vi "Climber Controller.vi"(8 "error in":errorcluster) -> ()   [LabVIEW 2019]
doc: "This VI executes continuously carrying out the current operation and responding to updates or new operations. It will often contain the timing or control code that is difficult to place directly in TeleOp. This VI generally opens all sensors and motors and isolates the rest of the robot code from knowing how the operations are carried out."
uses:
  Climber Setpoints.ctl
  Climber Operations.ctl
  <vilib>/Rock Robotics/WPI/Solenoid/WPI_SolenoidChannel.ctl
  <vilib>/Rock Robotics/WPI/Solenoid/WPI_SolenoidValue.ctl
  <vilib>/Rock Robotics/WPI/ThirdParty/Phoenix-LabVIEW/Motor Controller/Controls/CTRE_Phoenix_MotorControl_ControlMode.ctl
  <vilib>/Rock Robotics/WPI/ThirdParty/Phoenix-LabVIEW/Motor Controller/Controls/CTRE_Phoenix_MotorControl_NeutralMode.ctl
  <vilib>/Rock Robotics/WPI/Solenoid/WPI_SolenoidOpenSingle.vi
  <vilib>/Rock Robotics/WPI/Solenoid/WPI_SolenoidSetEnum.vi
  <vilib>/addons/control/pid/pid.llb/PID (DBL).vi
  <vilib>/Rock Robotics/Network Tables/NT Write Boolean.vi
  <vilib>/addons/control/pid/NI_PID_pid.lvlib
panel:
  out "Current\nCmd":string
  # "Tip: It may be helpful to observe inputs and sensor values.\nYou may also want to display tuning or debugging controls."
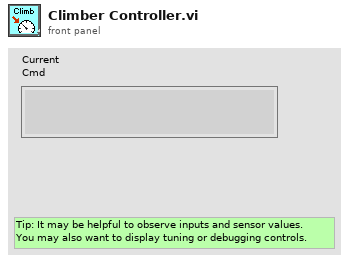
[diagram p1: front panel]
types:
  T1 = typedef "CTRE_Phoenix_MotorControl_NeutralMode.ctl" = enum8{"EEPROMSetting", "Override to Coast", "Override to Brake"}
  T2 = typedef "CTRE_Phoenix_MotorControl_ControlMode.ctl" = u16
  T3 = typedef "WPI_SolenoidValue.ctl" = enum16{"Off", "On", "Forward", "Reverse"}
  T4 = typedef "WPI_SolenoidChannel.ctl" = enum8{"Solenoid 0", "Solenoid 1", "Solenoid 2", "Solenoid 3", "Solenoid 4", "Solenoid 5", "Solenoid 6", "Solenoid 7", "Invalid"}
  T5 = typedef "Climber Setpoints.ctl" = cluster{"Operation":T6, "Setpoint":dbl, "Duration":dbl}
  T6 = typedef "Climber Operations.ctl" = enum16{"Reserve", "Read Current", "Immediate", "Up", "Down", "Position Auto", "Position Manual"}
  T7 = typedef "WPI_MotorControlDeviceRef.ctl" = cluster{"DeviceStatus":errorcluster, "Type":T8, "PWM":cluster{"PWM Channel":T9, "DeadBand":T10}, "CAN":cluster{"Device Number":u8, "SetOutput VI Ref":variant, "GetOutput VI Ref":variant, "Enable VI Ref":variant, "Disable VI Ref":variant, "Data":variant}, "Invert":bool, "DIO PWM":cluster{"PWM \"Enable\" Channel":T9, "DIOChannel":T11, "PWM Rate":dbl}}
  T8 = typedef "WPI_MotorControlType.ctl" = enum16{"PWM", "CAN", "DIO PWM"}
  T9 = typedef "FPGA_DIOPWMChannel.ctl" = enum8{"PWM 0", "PWM 1", "PWM 2", "PWM 3", "PWM 4", "PWM 5", "PWM 6", "PWM 7", "PWM 8", "PWM 9", "PWM MXP 0", "PWM MXP 1", "PWM MXP 2", "PWM MXP 3", "PWM MXP 4", "PWM MXP 5", "PWM MXP 6", "PWM MXP 7", "PWM MXP 8", "PWM MXP 9", "Invalid"}
  T10 = typedef "WPI_PWMDeadband.ctl" = cluster{"Name":string, "maxPositivePwm":i32, "minPositivePwm":i32, "centerPwm":i32, "maxNegativePwm":i32, "minNegativePwm":i32, "angularRange":u16}
  T11 = typedef "FPGA_DIOChannel.ctl" = enum8{"DIO 0", "DIO 1", "DIO 2", "DIO 3", "DIO 4", "DIO 5", "DIO 6", "DIO 7", "DIO 8", "DIO 9", "DIO MXP 0", "DIO MXP 1", "DIO MXP 2", "DIO MXP 3", "DIO MXP 4", "DIO MXP 5", "DIO MXP 6", "DIO MXP 7", "DIO MXP 8", "DIO MXP 9", "DIO MXP 10", "DIO MXP 11", "DIO MXP 12", "DIO MXP 13", "DIO MXP 14", "DIO MXP 15", "SPI Port CS1", "SPI Port CS2", "SPI Port CS3", "SPI Port MISO", "SPI Port MOSI", "Invalid"}
  T12 = typedef "WPI_SolenoidDevRef.ctl" = cluster{"DevStatus":errorcluster, "Pneumatics Control Module":u8, "Forward Solenoid Channel":T4, "Reverse Solenoid Channel":T4}
  T13 = typedef "Command Status Info.ctl" = cluster{"Name":string, "Status":T14, "notifier out":T15}
  T14 = typedef "Completion Status.ctl" = enum16{"Successful", "Aborted", "Incomplete"}
  T15 = typedef "Completion Notifier.ctl" = refnum<notifier>
  T16 = cluster{"Current Command":T5, "Command Timing":cluster{"Start Time (ms)":u32, "Iterations":i32}, "Command Arguments":cluster{"Command Info":T13, "Description":string, "Default Command":T5, "queue out":refnum<queue>, "Subsystem Name":string}}
  T17 = cluster{"proportional gain (Kc)":dbl, "integral time (Ti, min)":dbl, "derivative time (Td, min)":dbl}
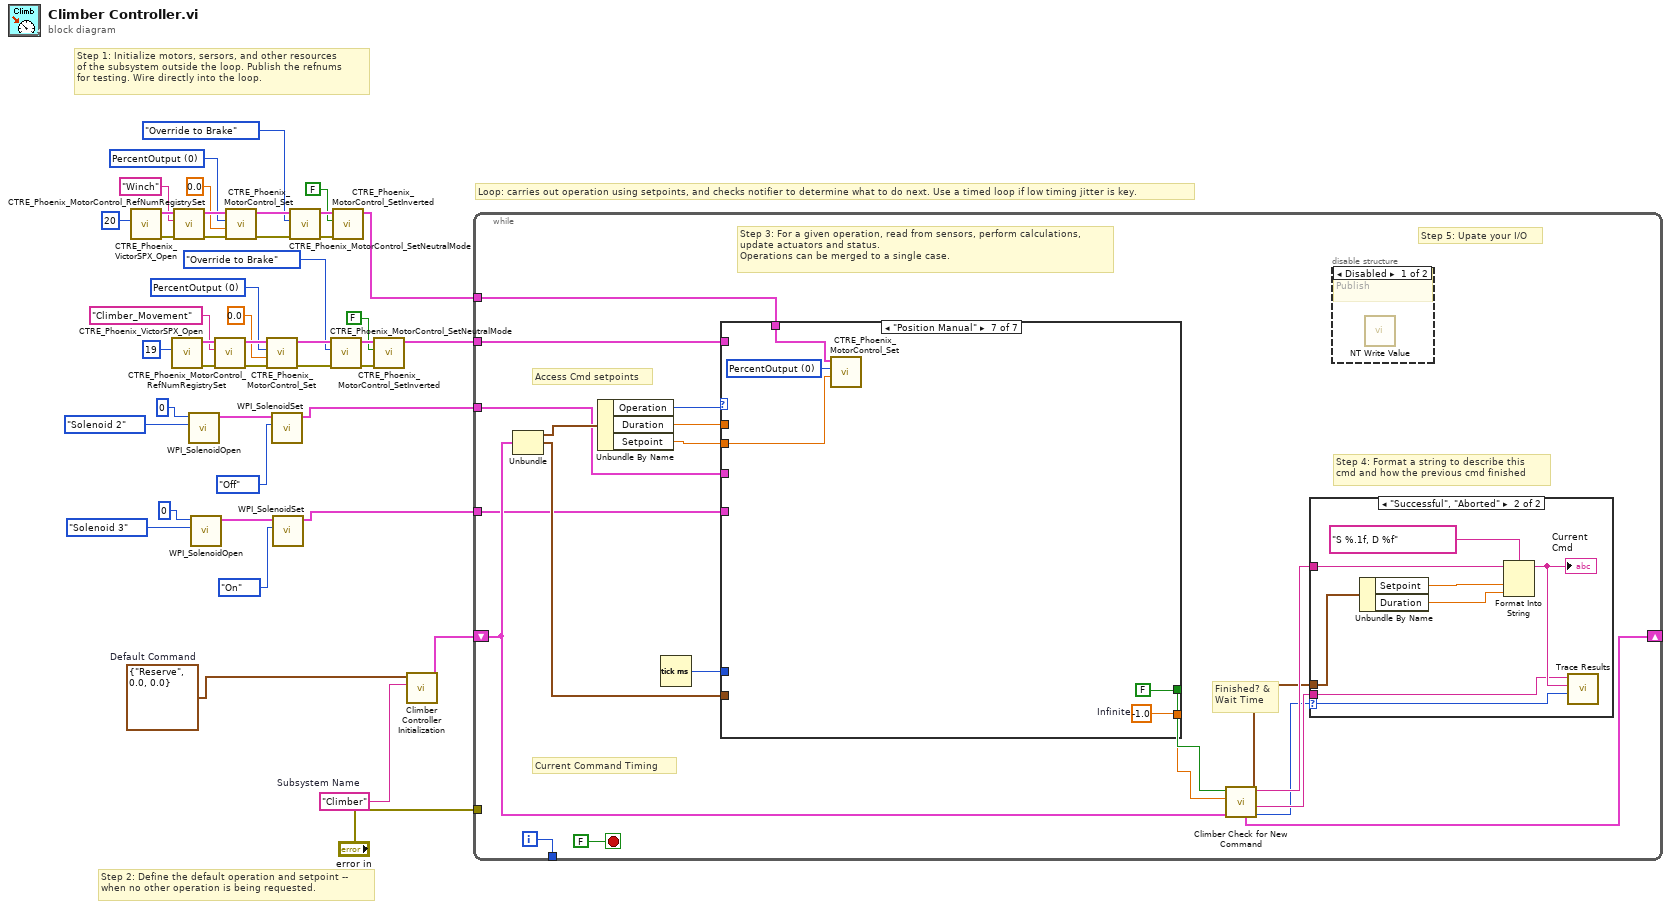
[diagram p0: block diagram]
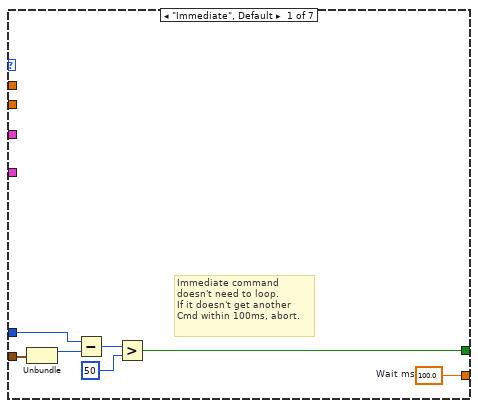
[diagram p4: hidden frame]
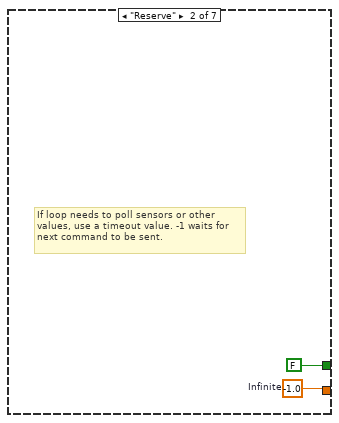
[diagram p5: hidden frame]
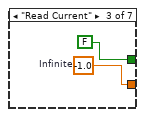
[diagram p6: hidden frame]
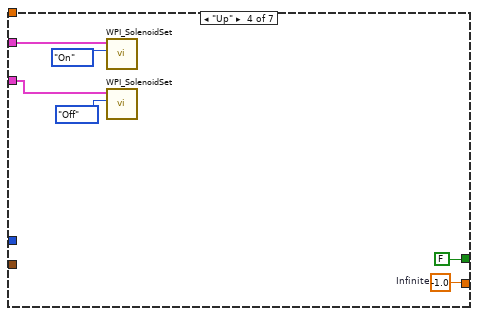
[diagram p7: hidden frame]
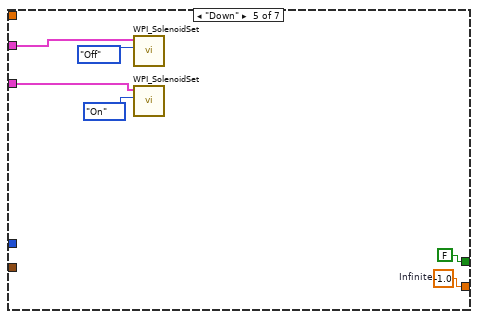
[diagram p8: hidden frame]
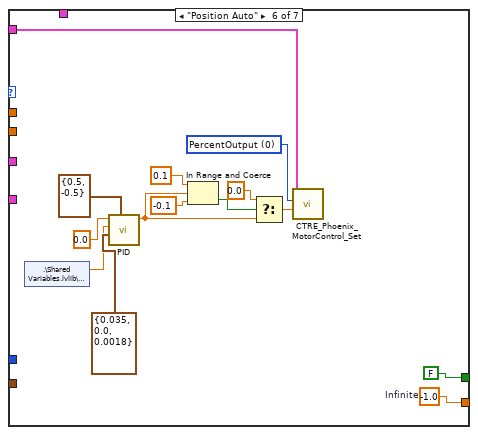
[diagram p9: hidden frame]
diagram:
  w6 = T2 0 items=["PercentOutput"=0, "Position"=1, "Velocity"=2, "Current"=3, "Follower"=5, "MotionProfile"=6, "MotionMagic"=7, "MotionProfileArc"=10, "Disabled"=15] ("Control Mode")
  w31 = T2 0 items=["PercentOutput"=0, "Position"=1, "Velocity"=2, "Current"=3, "Follower"=5, "MotionProfile"=6, "MotionMagic"=7, "MotionProfileArc"=10, "Disabled"=15] ("Control Mode")
  w41 = T5 {"Operation"=enum."Reserve", "Setpoint"=0.0, "Duration"=0.0}  # Default Command
  w42 = "Climber"  # Subsystem Name
  # "Step 2: Define the default operation and setpoint --\nwhen no other operation is being requested."
  # "Step 1: Initialize motors, sersors, and other resources\nof the subsystem outside the loop. Publish the refnums\nfor testing. Wire directly into the loop."
  # "Loop: carries out operation using setpoints, and checks notifier to determine what to do next. Use a timed loop if low timing jitter is key."
  n1 = call <vilib>:"CTRE_Phoenix_VictorSPX_Open.vi"("Device Number"=u8 20) -> ("error out"=w8:errorcluster, "CAN Talon SRX Ref"=w15:T7)  [unwired: 9 in]
  n2 = call <vilib>:"CTRE_Phoenix_VictorSPX_Open.vi"("Device Number"=u8 19) -> ("error out"=w33:errorcluster, "CAN Talon SRX Ref"=w40:T7)  [unwired: 9 in]
  n3 = call <vilib>:"CTRE_Phoenix_MotorControl_RefNumRegistrySet.vi"("error in (no error)"=w8, "refnum name"="Winch", "PhoenixMotorControlDevRef"=w15) -> ("error out"=w9:errorcluster, "PhoenixMotorControlDevRef"=w14:T7)  [unwired: 7 in]
  n4 = call-poly <vilib>:"WPI_SolenoidOpen.vi"("Solenoid Channel"=WPI_SolenoidChannel."Solenoid 2", "Pneumatics Control Module (0)"=u8 0) -> ("SolenoidDevRef"=w18:T12)  [unwired: 8 in, 1 out]
  n5 = call-poly <vilib>:"WPI_SolenoidOpen.vi"("Solenoid Channel"=WPI_SolenoidChannel."Solenoid 3", "Pneumatics Control Module (0)"=u8 0) -> ("SolenoidDevRef"=w16:T12)  [unwired: 8 in, 1 out]
  n6 = call <vilib>:"CTRE_Phoenix_MotorControl_RefNumRegistrySet.vi"("error in (no error)"=w33, "refnum name"="Climber_Movement", "PhoenixMotorControlDevRef"=w40) -> ("error out"=w34:errorcluster, "PhoenixMotorControlDevRef"=w39:T7)  [unwired: 7 in]
  n7 = call <vilib>:"CTRE_Phoenix_MotorControl_Set.vi"("error in (no error)"=w9, "Output"=0.0, "Control Mode"=w6, "PhoenixMotorControlDevRef"=w14) -> ("error out"=w10:errorcluster, "PhoenixMotorControlDevRef"=w13:T7)  [unwired: 6 in]
  n8 = call <vilib>:"CTRE_Phoenix_MotorControl_Set.vi"("error in (no error)"=w34, "Output"=0.0, "Control Mode"=w31, "PhoenixMotorControlDevRef"=w39) -> ("error out"=w35:errorcluster, "PhoenixMotorControlDevRef"=w38:T7)  [unwired: 6 in]
  n9 = call-poly <vilib>:"WPI_SolenoidSet.vi"("Value"=WPI_SolenoidValue."Off", "SolenoidDevRef"=w18) -> ("SolenoidDevRef"=w19:T12)  [unwired: 8 in, 1 out]
  n10 = call-poly <vilib>:"WPI_SolenoidSet.vi"("Value"=WPI_SolenoidValue."On", "SolenoidDevRef"=w16) -> ("SolenoidDevRef"=w17:T12)  [unwired: 8 in, 1 out]
  n11 = call <vilib>:"CTRE_Phoenix_MotorControl_SetNeutralMode.vi"("error in (no error)"=w10, "Motor Control Neutral Mode"=CTRE_Phoenix_MotorControl_NeutralMode."Override to Brake", "PhoenixMotorControlDevRef"=w13) -> ("error out"=w11:errorcluster, "PhoenixMotorControlDevRef"=w12:T7)  [unwired: 7 in]
  n12 = call <vilib>:"CTRE_Phoenix_MotorControl_SetNeutralMode.vi"("error in (no error)"=w35, "Motor Control Neutral Mode"=CTRE_Phoenix_MotorControl_NeutralMode."Override to Brake", "PhoenixMotorControlDevRef"=w38) -> ("error out"=w36:errorcluster, "PhoenixMotorControlDevRef"=w37:T7)  [unwired: 7 in]
  n13 = call <vilib>:"CTRE_Phoenix_MotorControl_SetInverted.vi"("error in (no error)"=w11, "Invert?"=FALSE, "PhoenixMotorControlDevRef"=w12) -> ("PhoenixMotorControlDevRef"=w1:T7)  [unwired: 7 in, 1 out]
  n14 = call <vilib>:"CTRE_Phoenix_MotorControl_SetInverted.vi"("error in (no error)"=w36, "Invert?"=FALSE, "PhoenixMotorControlDevRef"=w37) -> ("PhoenixMotorControlDevRef"=w26:T7)  [unwired: 7 in, 1 out]
  n15 = call "Climber Controller Initialization.vi"("Subsystem Name"=w42, "Default Command"=w41) -> ("Current Command"=w43:T16)  [unwired: 9 in]
  n16 = while {
    shift-right: [w56] -> _
    shift-left: w43 -> [w49]
    tunnel: [w63] -> _
    tunnel: "error in" -> [_]
    tunnel: w26 -> [w48]
    tunnel: w17 -> [w47]
    tunnel: w19 -> [w46]
    tunnel: w1 -> [w45]
    i -> [w63]
    stop <- FALSE stop-if-true
    # "Step 5: Upate your I/O"
    # "Step 4: Format a string to describe this\ncmd and how the previous cmd finished"
    # "Current Command Timing"
    # "Access Cmd setpoints"
    # "Finished? &\nWait Time"
    # "Step 3: For a given operation, read from sensors, perform calculations,\nupdate actuators and status.\nOperations can be merged to a single case."
    n17 = Unbundle(w49) -> ("Current Command"=w62:T5, "Command Timing"=w58:cluster{"Start Time (ms)":u32, "Iterations":i32})  [unwired: 1 out]
    n18 = Unbundle By Name(w62) -> ("Operation"=w61:T6, "Duration"=w60:dbl, "Setpoint"=w57:dbl)
    n19 = Tick Count (ms)() -> (millisecond timer value=w59:u32)
    n20 = case shown="\"Position Manual\"" w61 {
      tunnel: [w79 w81 w82 w88 w94 w108 w113] -> w54
      tunnel: [w73 FALSE ("ignore previous (F)") FALSE ("ignore previous (F)") FALSE ("ignore previous (F)") FALSE ("ignore previous (F)") FALSE ("ignore previous (F)") FALSE ("ignore previous (F)")] -> w55
      tunnel: w58 -> [w75 _ _ _ _ _ _]
      tunnel: w60 -> [_ _ _ _ _ _ _]
      tunnel: w59 -> [w74 _ _ _ _ _ _]
      tunnel: w57 -> [_ _ _ _ _ _ w112]
      tunnel: w48 -> [_ _ _ _ _ w107 _]
      tunnel: w47 -> [_ _ _ w86 w91 _ _]
      tunnel: w46 -> [_ _ _ w87 w90 _ _]
      tunnel: w45 -> [_ _ _ _ _ _ w110]
      frame "Immediate", Default {
        w79 = 100.0  # Wait ms
        # "Immediate command\ndoesn't need to loop.\nIf it doesn't get another\nCmd within 100ms, abort."
        n21 = Unbundle(w75) -> ("Start Time (ms)"=w78:u32)  [unwired: 1 out]
        n22 = Subtract(x=w74, y=w78) -> (x-y=w77:u32)
        n23 = Greater?(x=w77, y=u8 50 ("Left Motor")) -> (0:w73:bool)
      }
      frame "Reserve" {
        w81 = -1.0  # Infinite
        # "If loop needs to poll sensors or other\nvalues, use a timeout value. -1 waits for\nnext command to be sent."
      }
      frame "Read Current" {
        w82 = -1.0  # Infinite
      }
      frame "Up" {
        w88 = -1.0  # Infinite
        n24 = call-poly <vilib>:"WPI_SolenoidSet.vi"("Value"=WPI_SolenoidValue."On", "SolenoidDevRef"=w87) -> ()  [unwired: 8 in, 2 out]
        n25 = call-poly <vilib>:"WPI_SolenoidSet.vi"("Value"=WPI_SolenoidValue."Off", "SolenoidDevRef"=w86) -> ()  [unwired: 8 in, 2 out]
      }
      frame "Down" {
        w94 = -1.0  # Infinite
        n26 = call-poly <vilib>:"WPI_SolenoidSet.vi"("Value"=WPI_SolenoidValue."Off", "SolenoidDevRef"=w90) -> ()  [unwired: 8 in, 2 out]
        n27 = call-poly <vilib>:"WPI_SolenoidSet.vi"("Value"=WPI_SolenoidValue."On", "SolenoidDevRef"=w91) -> ()  [unwired: 8 in, 2 out]
      }
      frame "Position Auto" {
        w96 = T2 0 items=["PercentOutput"=0, "Position"=1, "Velocity"=2, "Current"=3, "Follower"=5, "MotionProfile"=6, "MotionMagic"=7, "MotionProfileArc"=10, "Disabled"=15] ("Control Mode")
        w108 = -1.0  # Infinite
        n28 = shared-variable ".\\Shared Variables.lvlib\\Roll"() -> (w103:dbl)  [unwired: 1 in, 1 out]
        n29 = call-poly <vilib>:"PID.vi"("output range"=cluster{"output high":dbl, "output low":dbl} {"output high"=0.5, "output low"=-0.5}, "PID gains"=T17 {"proportional gain (Kc)"=0.035, "integral time (Ti, min)"=0.0, "derivative time (Td, min)"=0.0018}, "process variable"=w103, "setpoint"=0.0) -> ("output"=w98:dbl)  [unwired: 6 in, 1 out]
        n30 = In Range and Coerce(upper limit=0.1, x=w98, lower limit=-0.1) -> (In Range?=w100:bool)  [unwired: 1 out]
        n31 = Select(t=0.0, s=w100, f=w98) -> (s? t:f=w97:dbl)
        n32 = call <vilib>:"CTRE_Phoenix_MotorControl_Set.vi"("Output"=w97, "Control Mode"=w96, "PhoenixMotorControlDevRef"=w107) -> ()  [unwired: 7 in, 2 out]
      }
      frame "Position Manual" {
        w111 = T2 0 items=["PercentOutput"=0, "Position"=1, "Velocity"=2, "Current"=3, "Follower"=5, "MotionProfile"=6, "MotionMagic"=7, "MotionProfileArc"=10, "Disabled"=15] ("Control Mode")
        w113 = -1.0  # Infinite
        n33 = call <vilib>:"CTRE_Phoenix_MotorControl_Set.vi"("Output"=w112, "Control Mode"=w111, "PhoenixMotorControlDevRef"=w110) -> ()  [unwired: 7 in, 2 out]
      }
    }
    n34 = call "Climber Check for New Command.vi"("Current Command"=w49, "Wait time (ms)"=w54, "Finished?"=w55) -> ("Completion"=w50:T14, "Subsystem Name"=w51:string, "Current Command"=w52:T5, "Initial Trace String"=w53:string, "NextCommand"=w56:T16)  [unwired: 4 in]
    n35 = case shown="\"Successful\", \"Aborted\"" w50 {
      selector: w50 -> [_ w72]
      tunnel: w53 -> [_ w68]
      tunnel: w52 -> [_ w69]
      tunnel: w51 -> [_ w65]
      frame "Incomplete", Default {
        # "Continuing current command"
      }
      frame "Successful", "Aborted" {
        # "Report and setup for next command"
        n36 = Unbundle By Name(w69) -> ("Setpoint"=w71:dbl, "Duration"=w66:dbl)
        n37 = Format Into String(format string="S %.1f, D %f", initial string=w68, w71, w66) -> (resulting string=w67:string)  [unwired: 1 in, 1 out]
        "Current\nCmd" <- w67
        n38 = call <vilib>:"Trace Results.vi"("Status of previous command"=w72, "Description"=w67, "Subsystem"=w65) -> ()  [unwired: 9 in]
      }
    }
    n39 = disable-structure shown="Disabled" {
      frame Disabled {
        # "Publish"
        n40 = call-poly <vilib>:"NT Write Value.vi"() -> ()  [unwired: 11 in, 1 out]
      }
      frame Enabled {
      }
    }
  }
